vi "Shift_ABCD_SELECTION.vi"(7 "Where":string, 8 "error in (no error)":errorcluster, 9 "Array":string[](array[string]), 10 "table":string, 11 "Refnum in":T1) -> (0 "error out":errorcluster, 2 "Boolean":bool, 3 "Refnum out":T1)   [LabVIEW 2017]
uses:
  <vilib>/addons/database/Connection.llb/Conn ObjectReference.ctl
  <vilib>/addons/database/NI_Database_API.lvlib
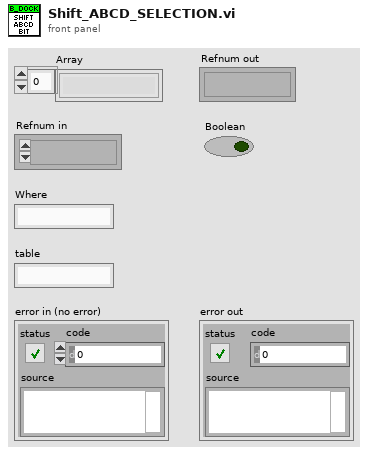
[diagram p1: front panel]
types:
  T1 = typedef "NI_Database_API.lvlib/Conn ObjectReference.ctl" = refnum<k1>
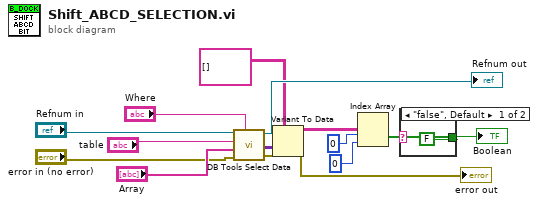
[diagram p0: block diagram]
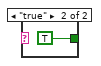
[diagram p2: hidden frame]
diagram:
  n1 = call <vilib>:"DB Tools Select Data.vi"("condition"="Where", "error in (no error)"="error in (no error)", "columns"="Array", "table"="table", "connection reference"="Refnum in") -> ("error out"=w6:errorcluster, "data"=w11:variant[][], "connection reference out"=→"Refnum out":T1)  [unwired: 1 in]
  n2 = Variant To Data(error in=w6, type=string[][] [], Variant=w11) -> (data=w8:string[][], error out=→"error out":errorcluster)
  n3 = Index Array(array=w8, index (row)=0, index (col)=0 ("disabled index (col)")) -> (element=w12:string)
  n4 = case shown="\"false\", Default" w12 {
    tunnel: [FALSE TRUE] -> w13
    frame "false", Default {
    }
    frame "true" {
    }
  }
  "Boolean" <- w13
